vi "DAQ - 15A.vi"(8 "error in":errorcluster, 11 "task out":refnum<k21>) -> (0 "error out":errorcluster, 2 "15A?":bool, 3 "task out":refnum<k21>)   [LabVIEW 2024]
doc: "Looking for voltage on this line using a 6525 DAQ. \nIf there is no 24V the loop will time out at 10 seconds.\nLink to start / end channel Vis.\nLooking at 15A connector"
uses:
  <vilib>/DAQmx/read.llb/DAQmx Read (Digital 1D Bool 1Chan 1Samp).vi
  <vilib>/DAQmx/miscellaneous.llb/DAQmx Fill In Error Info.vi
panel:
  out "Elapsed Time":dbl=1653.7379999160767
  out "DAQ Read 1":bool[](array[boolean])
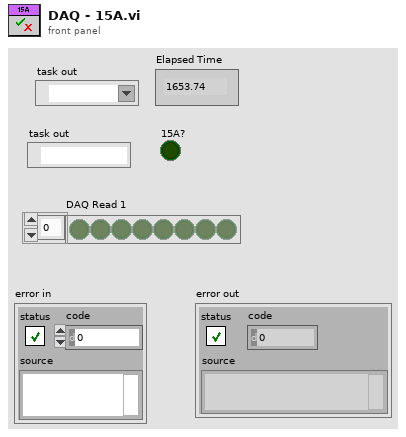
[diagram p1: front panel]
types:
  T1 = enum16{"Start Timer", "Get Time", "Pause", "Unpause"}
  T2 = cluster{"[0]":bool, "[1]":bool, "[2]":bool, "[3]":bool, "[4]":bool, "[5]":bool, "[6]":bool, "[7]":bool, "[8]":bool}
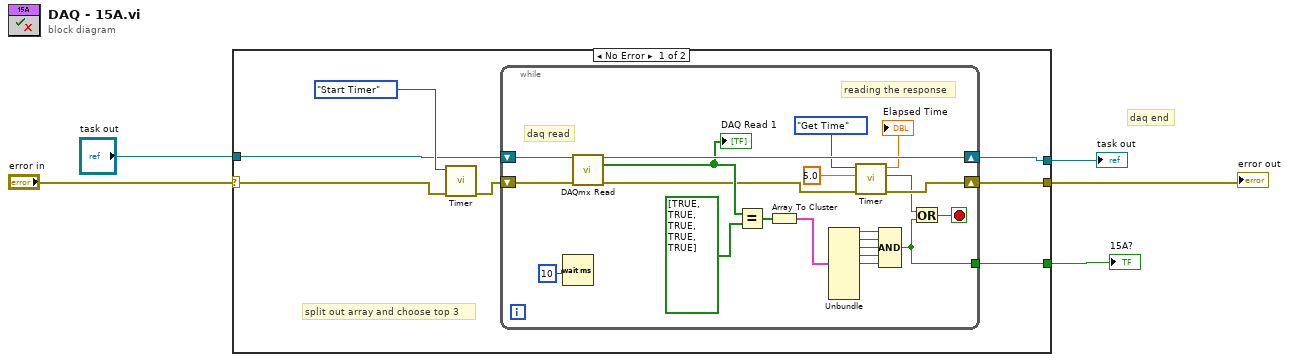
[diagram p0: block diagram]
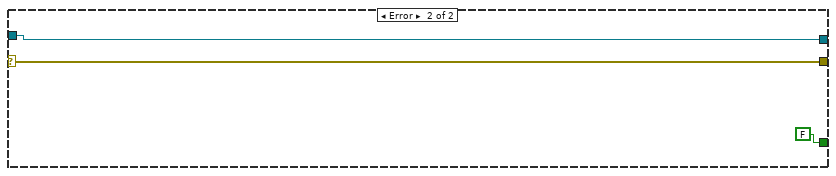
[diagram p2: hidden frame]
diagram:
  # "daq end"
  n1 = case shown="No Error" "error in" {
    selector: "error in" -> [w9 w35]
    tunnel: [w12 FALSE] -> w5
    tunnel: "task out" -> [w8 w36]
    tunnel: [w7 w36] -> w3
    tunnel: [w6 w35] -> w2
    frame No Error {
      # "split out array and choose top 3"
      n2 = call "Timer.vi"("error in (no error)"=w9, "Enum"=T1."Start Timer") -> ("error out"=w10:errorcluster)  [unwired: 6 in, 3 out]
      n3 = while {
        shift-right: [w32] -> w7
        shift-left: w8 -> [w33]
        shift-right: [w21] -> w6
        shift-left: w10 -> [w31]
        tunnel: [w20] -> w12
        stop <- w25 stop-if-true
        # "reading the response"
        # "daq read"
        n4 = Wait (ms)(milliseconds to wait=u32 10) -> ()  [unwired: 1 out]
        n5 = call-poly <vilib>:"DAQmx Read.vi"("task/channels in"=w33, "error in"=w31) -> ("task out"=w32:refnum<k21>, "data"=w27:bool[], "error out"=w22:errorcluster)  [unwired: 11 in]
        "DAQ Read 1" <- w27
        n6 = Equal?(x=w27, y=bool[] [TRUE, TRUE, TRUE, TRUE, TRUE] ("x")) -> (x = y?=w29:bool[])
        n7 = Array To Cluster(array=w29) -> (cluster=w28:T2)
        n8 = Unbundle(w28) -> ("[0]"=w26:bool, "[1]"=w17:bool, "[2]"=w15:bool, "[3]"=w14:bool, "[4]"=w13:bool)  [unwired: 4 out]
        n9 = call "Timer.vi"("error in (no error)"=w22, "Target Time"=5.0, "Enum"=T1."Get Time") -> ("error out"=w21:errorcluster, "Time Elapsed?"=w19:bool, "Elapsed Time"=→"Elapsed Time":dbl)  [unwired: 5 in, 1 out]
        n10 = Compound Arithmetic op=AND(w26, w17, w15, w14, w13) -> (w20:bool)
        n11 = Or(x=w19, y=w20) -> (x .or. y?=w25:bool)
      }
    }
    frame Error {
    }
  }
  "15A?" <- w5
  "error out" <- w2
  "task out" <- w3
